vi "ramp_09.vi"(0 "pause":bool=TRUE, 1 "manual":i32, 3 "T_man":dbl, 4 "Seq":dbl[](array[numeric])=[30.0, 50.0, 60.0, 30.0, 20.0], 5 "reset":bool, 6 "TimeParams":dbl[](array[numeric])=[1.0, 1.0, 1.0, 1.0, 1.0], 7 "shutdown":bool, 11 "port":i32=1, 12 "treshold":dbl) -> (9 "T in":dbl, 10 "STEP":i32, 13 "T ext":dbl, 14 "params":i32[](array[numeric]), 15 "T control":dbl)   [LabVIEW 2015]
uses:
  x64/Debug/BERTTA.dll
panel:
  out "params2":i32
  out "params0":i32
  out "params1":i32
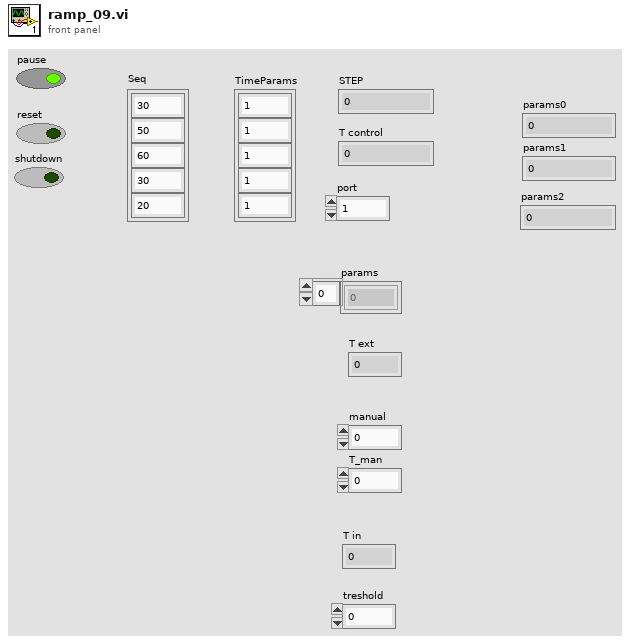
[diagram p1: front panel]
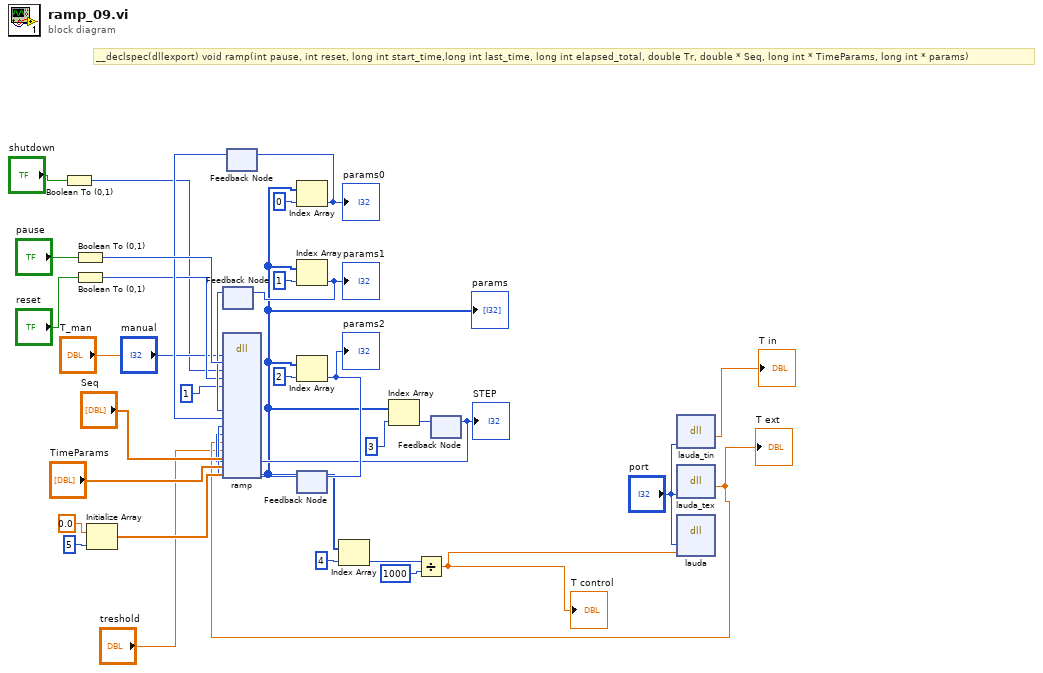
[diagram p0: block diagram]
diagram:
  # "__declspec(dllexport) void ramp(int pause, int reset, long int start_time,long int last_time, long int elapsed_total, double Tr, double * Seq, long int * TimeParams, long int * params)"
  n1 = Boolean To (0,1)(Boolean="shutdown") -> (0, 1=w1:i16)
  n2 = Boolean To (0,1)(Boolean="pause") -> (0, 1=w28:i16)
  n3 = Boolean To (0,1)(Boolean="reset") -> (0, 1=w22:i16)
  n4 = Initialize Array(0.0 ("element"), 5 ("dimension size")) -> (w35:dbl[])
  n5 = feedback #1() -> (w24:i32)  [unwired: 1 in]
  n6 = feedback #2() -> (w25:i32)  [unwired: 1 in]
  n7 = feedback #3() -> (w19:i32)  [unwired: 1 in]
  n8 = feedback #4() -> (w15:i32)  [unwired: 1 in]
  "STEP" <- w15
  n9 = dll-call lib="C:/Users/shresplab/OneDrive - Kemira Oyj/Documents/Visual Studio 2017/Projects/Bertta/BERTTA/x64/Debug/BERTTA.dll" fn="lauda_tin"("port"="port") -> ("return type"=→"T in":dbl)  [unwired: 4 in, 2 out]
  n10 = dll-call lib="C:/Users/shresplab/OneDrive - Kemira Oyj/Documents/Visual Studio 2017/Projects/Bertta/BERTTA/x64/Debug/BERTTA.dll" fn="lauda_tex"("port"="port") -> ("return type"=w8:dbl)  [unwired: 4 in, 2 out]
  "T ext" <- w8
  n11 = dll-call lib="C:/Users/shresplab/OneDrive - Kemira Oyj/Documents/Visual Studio 2017/Projects/Bertta/BERTTA/x64/Debug/BERTTA.dll" fn="ramp"("pause"=w28, "shutdown"=w1, "reset"=w22, "grad"=1, "manual"="manual", "T_man"="T_man", "start_time"=w24, "last_time"=w25, "elapsed_total"=w19, "step"=w15, "Tr"=w8, "treshold"="treshold", "Seq"="Seq", "TimeParams"="TimeParams", "params"=w35) -> ("params"=w11:i32[])  [unwired: 18 in, 2 out]
  "params" <- w11
  n12 = Index Array(array=w11, index=0) -> (element=w30:i32)
  "params0" <- w30
  n13 = feedback-in #2(w30) -> ()
  n14 = Index Array(array=w11, index=1) -> (element=w29:i32)
  "params1" <- w29
  n15 = feedback-in #1(w29) -> ()
  n16 = Index Array(array=w11, index=2) -> (element=w18:i32)
  "params2" <- w18
  n17 = feedback-in #3(w18) -> ()
  n18 = Index Array(array=w11, index=4) -> (element=w10:i32)
  n19 = Index Array(array=w11, index=3) -> (element=w16:i32)
  n20 = Divide(x=w10, y=1000) -> (x/y=w7:dbl)
  "T control" <- w7
  n21 = feedback-in #4(w16) -> ()
  n22 = dll-call lib="C:/Users/shresplab/OneDrive - Kemira Oyj/Documents/Visual Studio 2017/Projects/Bertta/BERTTA/x64/Debug/BERTTA.dll" fn="lauda"("port"="port", "set_temp"=w7) -> ()  [unwired: 6 in, 2 out]
